vi "Get all Object Items.vi"(8 "error in (no error)":errorcluster, 10 "Offset":i32, 11 "JSON":string) -> (0 "error out":errorcluster, 1 "<JSON>":string[](array[string]) caption="<JSON>Items", 2 "Offset past":i32 caption="Offset past Object", 3 "Item Names":string[](array[string]))   [LabVIEW 2017, in "JSONtext.lvlib"]
doc: "Return all Items in the Object as an array of JSON Values."
uses:
  JSONtext.lvlib
  Parsing/Parsing State.ctl
  Parsing/Advance past Number.vi
  support/Unescape JSON string.vi
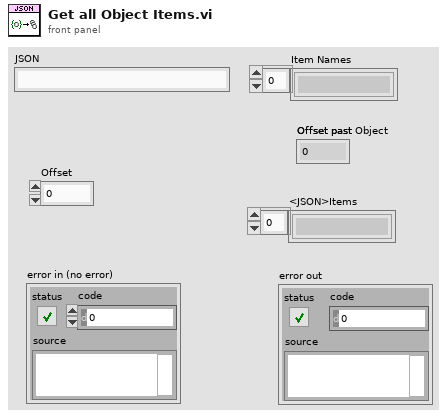
[diagram p1: front panel]
types:
  T1 = typedef "JSONtext.lvlib/Parsing State.ctl" = enum16{"Parser Error", "Object", "Array", "String", "Number/Other", "Leading Whitespace", "Object end", "Array end", "Value end"}
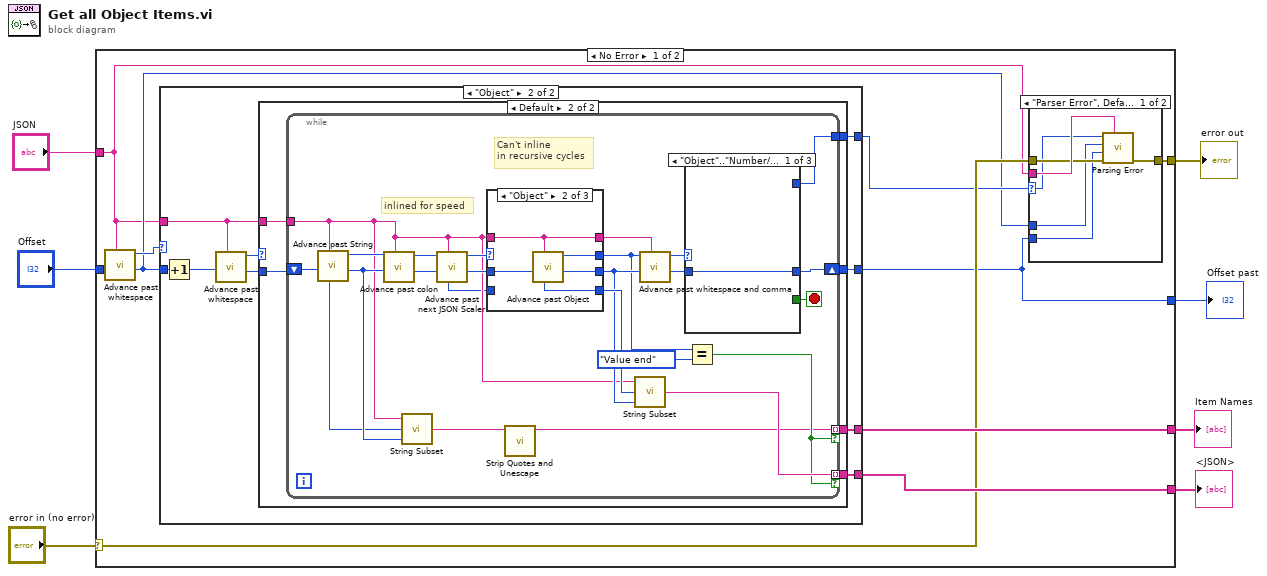
[diagram p0: block diagram]
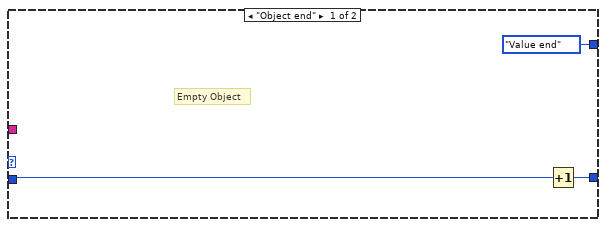
[diagram p3: hidden frame]
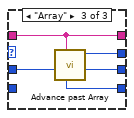
[diagram p5: hidden frame]
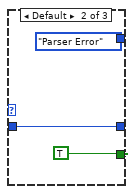
[diagram p6: hidden frame]
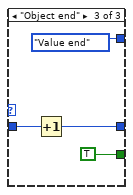
[diagram p7: hidden frame]
diagram:
  n1 = case shown="No Error" "error in (no error)" {
    selector: "error in (no error)" -> [w12 w92]
    tunnel: [w17 _] -> w7
    tunnel: [w16 _] -> w6
    tunnel: "Offset" -> [w15 w91]
    tunnel: [w13 w92] -> w4
    tunnel: [w11 w91] -> w2
    tunnel: "JSON" -> [w8 _]
    frame No Error {
      n2 = call "Advance past whitespace.vi"("JSON"=w8, "Offset"=w15) -> ("Offset of first non-whitespace"=w9:i32, "Parser State"=w14:T1)  [unwired: 8 in]
      n3 = case shown="\"Object\"" w14 {
        selector: w14 -> [w19 _]
        tunnel: [w19 w28] -> w10
        tunnel: [_ w27] -> w17
        tunnel: [_ w26] -> w16
        tunnel: w9 -> [w18 w25]
        tunnel: w8 -> [_ w21]
        tunnel: [w18 w24] -> w11
        frame "Parser Error", Default {
        }
        frame "Object" {
          n4 = Increment(x=w25) -> (x+1=w23:i32)
          n5 = call "Advance past whitespace.vi"("JSON"=w21, "Offset"=w23) -> ("Offset of first non-whitespace"=w22:i32, "Parser State"=w20:T1)  [unwired: 8 in]
          n6 = case shown="Default" w20 {
            tunnel: [Parsing_State."Value end" w37] -> w28
            tunnel: [_ w36] -> w27
            tunnel: [_ w35] -> w26
            tunnel: [w30 w34] -> w24
            tunnel: w22 -> [w29 w33]
            tunnel: w21 -> [_ w32]
            frame "Object end" {
              # "Empty Object"
              n7 = Increment(x=w29) -> (x+1=w30:i32)
            }
            frame Default {
              n8 = while {
                shift-right: [w58] -> w34
                shift-left: w33 -> [w38]
                tunnel: w32 -> [w47]
                tunnel: [w56] -> w37
                tunnel: [w41] -> w36 mode=indexing if=w43
                tunnel: [w46] -> w35 mode=indexing if=w43
                stop <- w57 stop-if-true
                # "Can't inline\nin recursive cycles"
                # "inlined for speed"
                n9 = call "Advance past String.vi"("JSON"=w47, "Offset"=w38) -> ("Offset past match"=w50:i32, "State"=w61:T1, "Value start out"=w40:i32)  [unwired: 7 in]
                n10 = call "Advance past colon.vi"("JSON"=w47, "Offset"=w50, "State"=w61) -> ("index"=w52:i32, "State"=w53:T1)  [unwired: 7 in]
                n11 = call "String Subset.vi"("Offset past End"=w50, "Start offset"=w40, "JSON"=w47) -> ("substring"=w42:string)  [unwired: 2 in]
                n12 = call "Advance past next JSON Scaler.vi"("JSON"=w47, "Offset"=w52, "Parser State in"=w53) -> ("index"=w51:i32, "Parser State"=w54:T1, "Value start"=w39:i32)  [unwired: 6 in]
                n13 = case shown="\"Object\"" w54 {
                  selector: w54 -> [w64 _ _]
                  tunnel: w51 -> [w63 w70 w75]
                  tunnel: [w64 w69 w74] -> w45
                  tunnel: [w63 w68 w73] -> w48
                  tunnel: w47 -> [w65 w67 w72]
                  tunnel: [w65 w67 w72] -> w55
                  tunnel: [w62 w66 w71] -> w49
                  tunnel: w39 -> [w62 _ _]
                  frame Default {
                  }
                  frame "Object" {
                    n14 = call "Advance past Object.vi"("JSON"=w67, "Offset"=w70) -> ("Offset past Object"=w68:i32, "State"=w69:T1, "Object Start"=w66:i32)  [unwired: 7 in]
                  }
                  frame "Array" {
                    n15 = call "Advance past Array.vi"("JSON"=w72, "Offset"=w75) -> ("Offset past Array"=w73:i32, "State"=w74:T1, "Array Start"=w71:i32)  [unwired: 7 in]
                  }
                }
                n16 = call "Strip Quotes and Unescape.vi"("String"=w42) -> ("result string"=w41:string)  [unwired: 9 in, 1 out]
                n17 = call "String Subset.vi"("Offset past End"=w48, "Start offset"=w49, "JSON"=w47) -> ("substring"=w46:string)  [unwired: 2 in]
                n18 = call "Advance past whitespace and comma.vi"("JSON"=w55, "Offset"=w48, "State in"=w45) -> ("Offset past match"=w60:i32, "State"=w59:T1)  [unwired: 7 in]
                n19 = case shown="\"Object\"..\"Number/Other\"" w59 {
                  tunnel: [_ TRUE TRUE] -> w57
                  tunnel: [_ Parsing_State."Parser Error" Parsing_State."Value end"] -> w56
                  tunnel: w60 -> [w76 w77 w81]
                  tunnel: [w76 w77 w80] -> w58
                  frame "Object".."Number/Other" {
                  }
                  frame Default {
                  }
                  frame "Object end" {
                    n20 = Increment(x=w81) -> (x+1=w80:i32)
                  }
                }
                n21 = Equal?(x=w45, y=Parsing_State."Value end") -> (x = y?=w43:bool)
              }
            }
          }
        }
      }
      n22 = case shown="\"Parser Error\", Default" w10 {
        selector: w10 -> [w84 _]
        tunnel: w8 -> [w89 _]
        tunnel: w12 -> [w88 w90]
        tunnel: [w87 w90] -> w13
        tunnel: w9 -> [w86 _]
        tunnel: w11 -> [w85 _]
        frame "Parser Error", Default {
          n23 = call "Parsing Error.vi"("JSON"=w89, "error in (no error)"=w88, "Offset past match"=w85, "Value start"=w86, "State"=w84) -> ("error out"=w87:errorcluster)  [unwired: 6 in]
        }
        frame "Value end" {
        }
      }
    }
    frame Error {
    }
  }
  "Item Names" <- w7
  "<JSON>" <- w6
  "error out" <- w4
  "Offset past" <- w2
